vi "运维调试_其他.vi"() -> ()   [LabVIEW 2016, in "其他.lvlib"]
uses:
  <vilib>/Utility/miscctls.llb/LVPointTypeDef.ctl
  PLC/PLC.lvlib
panel:
  out "集成报警信息":string
  out "R115":i16 caption="灯带关闭时间"
  out "R114":i16 caption="灯带开启时间"
  in  "照明":bool
  in  "侧边灯带":bool
  # "H"
  # "H"
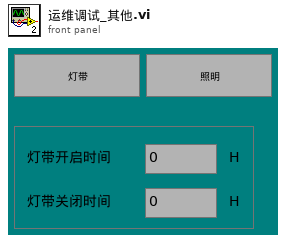
[diagram p1: front panel]
types:
  T1 = cluster{"R100":i16, "R101":i16, "R102":i16, "R103":i16, "R104":i16, "R105":i16, "R106":i16, "R107":i16, "R108":i16, "R109":i16, "R110":i16, "R111":i16, "R112":i16, "R113":i16, "R114":i16, "R115":i16, "R116":i16, "R117":i16, "R118":i16, "R119":i16, "R120":i16, "R121":i16, "R122":i16, "R123":i16, "R124":i16}
  T2 = typedef "LVPointTypeDef.ctl" = cluster{"Horizontal":i16, "Vertical":i16}
  T3 = cluster{"命令":string, "data":cluster{"starting address":u16, "coil values":bool[]}}
  T4 = cluster{"命令":string, "数据":cluster{"starting address":u16, "holding register values":u16[]}}
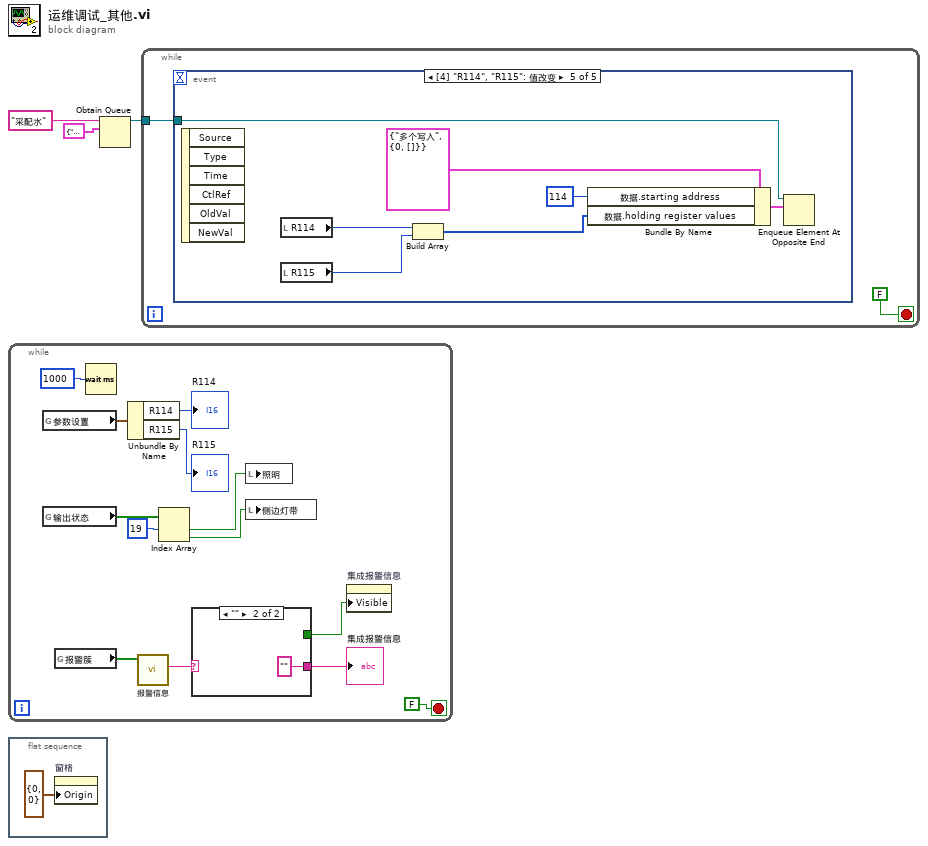
[diagram p0: block diagram]
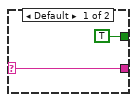
[diagram p2: hidden frame]
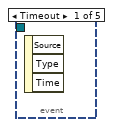
[diagram p3: hidden frame]
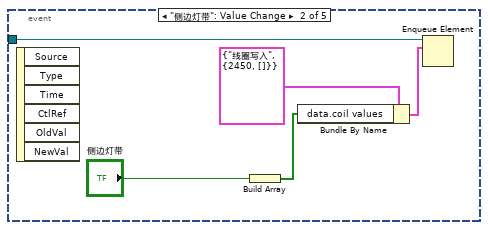
[diagram p4: hidden frame]
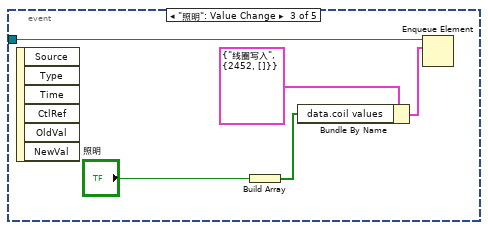
[diagram p5: hidden frame]
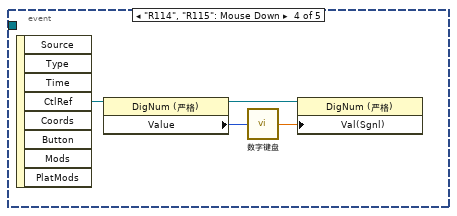
[diagram p6: hidden frame]
diagram:
  n1 = while {
    stop <- FALSE stop-if-true
    n2 = global read "采配水全局变量.vi" "参数设置"() -> (w14:T1)
    n3 = global read "采配水全局变量.vi" "输出状态"() -> (w7:bool[])
    n4 = global read "采配水全局变量.vi" "报警簇"() -> (w8:bool[])
    n5 = Wait (ms)(milliseconds to wait=u32 1000 ("等待时间（毫秒）")) -> ()  [unwired: 1 out]
    n6 = Unbundle By Name(w14) -> ("R114"=→"R114":i16, "R115"=→"R115":i16)
    n7 = call "报警信息.vi"("报警簇"=w8) -> ("系统报警信息"=w11:string)  [unwired: 9 in, 1 out]
    n8 = Index Array(array=w7, index #1=19 ("索引")) -> (element #1=w6:bool, element #2=w5:bool)  [unwired: 1 in]
    n9 = case shown="\"\"" w11 {
      selector: w11 -> [w18 _]
      tunnel: [w18 "" ("字符串")] -> w9
      tunnel: [TRUE ("可见") _] -> w10
      frame Default {
      }
      frame "" {
      }
    }
    "集成报警信息" <- w9
    n10 = local write "照明"(w6) -> ()
    n11 = local write "侧边灯带"(w5) -> ()
    n12 = property on="集成报警信息" class="Str"("Visible"=w10) -> ()  [unwired: 2 in, 2 out]
  }
  n13 = flat-sequence {
    frame #0 {
      n14 = property on="窗格" class="Pane"("Origin"=T2 {"Horizontal"=0, "Vertical"=0} ("原点")) -> ()  [unwired: 2 in, 2 out]
    }
  }
  n15 = Obtain Queue(name (unnamed)="采配水" ("名称（未命名）"), element data type=cluster{"命令":string, "数据":variant} {"命令"="", "数据"=variant}) -> (queue out=w1:refnum<queue>)  [unwired: 3 in, 2 out]
  n16 = while {
    tunnel: w1 -> [w21]
    stop <- FALSE stop-if-true
    n17 = event shown="[4] \"R114\", \"R115\": 值改变" {
      selector: _ -> [_ _ _ _ _]
      dyn-events: _ -> [_ _ _ _ _]
      timeout: _ -> [_ _ _ _ _]
      tunnel: w21 -> [_ w24 w30 _ w37]
      event Timeout {
        n18 = event-data() -> ()  [unwired: 1 in, 3 out]
      }
      event "侧边灯带": Value Change {
        n19 = event-data() -> ()  [unwired: 1 in, 6 out]
        n20 = Build Array("侧边灯带") -> (w23:bool[])
        n21 = Bundle By Name(cluster=T3 {"命令"="线圈写入", "data"={"starting address"=2450, "coil values"=[]}} ("元素"), "data.coil values"=w23) -> (w25:T3)
        n22 = Enqueue Element(queue=w24, element=w25) -> ()  [unwired: 2 in, 3 out]
      }
      event "照明": Value Change {
        n23 = event-data() -> ()  [unwired: 1 in, 6 out]
        n24 = Build Array("照明") -> (w29:bool[])
        n25 = Bundle By Name(cluster=T3 {"命令"="线圈写入", "data"={"starting address"=2452, "coil values"=[]}} ("元素"), "data.coil values"=w29) -> (w31:T3)
        n26 = Enqueue Element(queue=w30, element=w31) -> ()  [unwired: 2 in, 3 out]
      }
      event "R114", "R115": Mouse Down {
        n27 = event-data() -> ("CtlRef"=w36:refnum<vi>)  [unwired: 1 in, 7 out]
        n28 = property class="DigNum (严格)"(reference=w36) -> (reference out=w35:refnum<vi>, "Value"=w34:i16)  [unwired: 1 in, 1 out]
        n29 = call "数字键盘.vi"("OldNumber"=w34) -> ("NewNumber"=w33:sgl)
        n30 = property class="DigNum (严格)"(reference=w35, "Val(Sgnl)"=w33) -> ()  [unwired: 1 in, 2 out]
      }
      event "R114", "R115": Value Change {
        n31 = event-data() -> ()  [unwired: 1 in, 6 out]
        n32 = local read "R114"() -> (w42:i16)
        n33 = local read "R115"() -> (w43:i16)
        n34 = Build Array(w42, w43) -> (w38:i16[])
        n35 = Bundle By Name(cluster=T4 {"命令"="多个写入", "数据"={"starting address"=0, "holding register values"=[]}} ("元素"), "数据.starting address"=u16 114, "数据.holding register values"=w38) -> (w39:T4)
        n36 = Enqueue Element At Opposite End(queue=w37, element=w39) -> ()  [unwired: 2 in, 3 out]
      }
    }
  }
